vi "Camera.SetSession.vi"(8 "error in (no error)":errorcluster, 9 "Image":T1, 10 "Session":T2="cam0", 11 "Camera.Simulated":refnum<class "Camera.IMAQdx.lvclass">) -> (0 "error out":errorcluster, 3 "Camera.Simulated":refnum<class "Camera.IMAQdx.lvclass">)   [LabVIEW 2020, in "Camera.IMAQdx.lvclass"]
doc: "---------------------------------------------------------------\nJKI State Machine Objects™\nhttp://jki.net/state-machine-objects/\nCopyright (C) 2005-2015, JKI <info@jki.net>\nALL RIGHTS RESERVEDJKI State Machine Objects (SMO) 1.0.0.4\nJKI - JKI\nCopyright (c) 2015, JKI"
uses:
  Camera.IMAQdx.lvclass
  <vilib>/userdefined/High Color/IMAQdx.ctl
  <vilib>/vision/Image Controls.llb/IMAQ Image.ctl
  Camera.IMAQdx.lvclass/Camera.IMAQdx.ctl
panel:
  # "For instructions on how to use the JKI State Machine Objects, examples and video tutorials, visit:\nhttp://jki.net/state-machine-objects/\n\nJKI State Machine Objects™\nhttp://jki.net/state-machine-objects/\nCopyright (C) 2005-2015, JKI <info@jki.net>\nALL RIGHTS RESERVED"
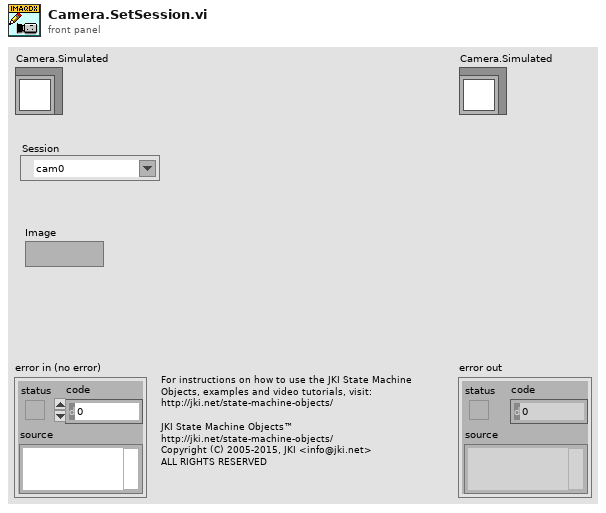
[diagram p1: front panel]
types:
  T1 = typedef "IMAQ Image.ctl" = refnum<image>
  T2 = typedef "IMAQdx.ctl" = refnum<k21>
  T3 = typedef "Camera.IMAQdx.lvclass/PrivateData--Ref.ctl" = refnum<data-value>
  T4 = typedef "Camera.IMAQdx.lvclass/PrivateData--Cluster.ctl" = cluster{"Session":T2, "Image":T1}
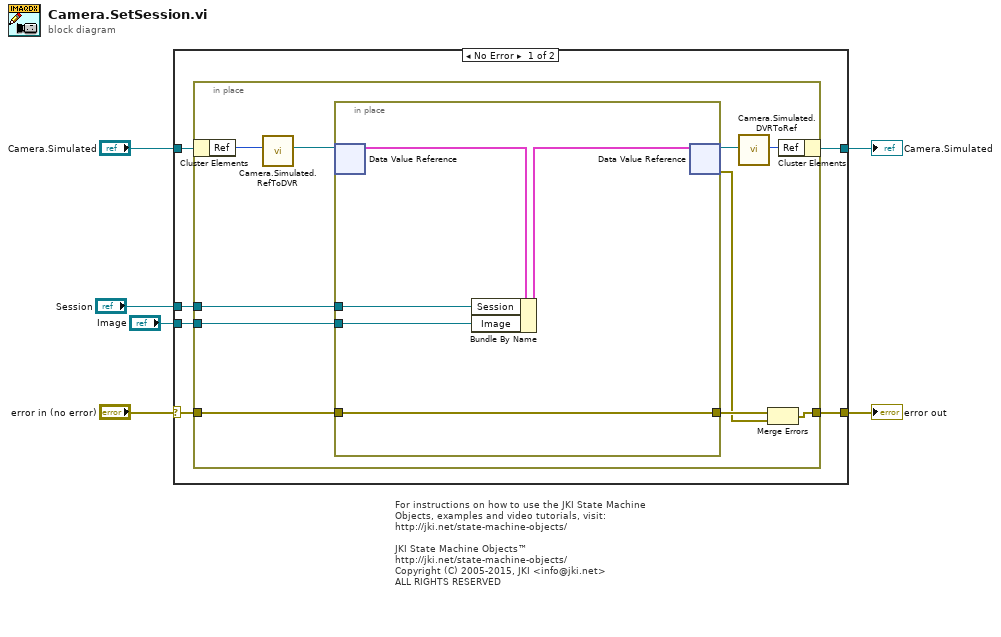
[diagram p0: block diagram]
diagram:
  # "For instructions on how to use the JKI State Machine Objects, examples and video tutorials, visit:\nhttp://jki.net/state-machine-objects/\n\nJKI State Machine Objects™\nhttp://jki.net/state-machine-objects/\nCopyright (C) 2005-2015, JKI <info@jki.net>\nALL RIGHTS RESERVED"
  n1 = case shown="No Error" "error in (no error)" {
    selector: "error in (no error)" -> [w10 w29]
    tunnel: [w9 w29] -> w5
    tunnel: [w11 w28] -> w6
    tunnel: "Camera.Simulated" -> [w12 w28]
    tunnel: "Session" -> [w8 _]
    tunnel: "Image" -> [w7 _]
    frame No Error {
      n2 = in-place {
        in-place-border: w10 -> [w22]
        in-place-border: [w19] -> w9
        in-place-border: w8 -> [w18]
        in-place-border: w7 -> [w13]
        n3 = in-place-cluster #1(w12) -> ("Ref"=w15:u32)
        n4 = call "Camera.Simulated.RefToDVR.vi"("Ref"=w15) -> ("Ref"=w14:T3)  [unwired: 10 in]
        n5 = in-place {
          in-place-border: w22 -> [w25]
          in-place-border: [w25] -> w21
          in-place-border: w18 -> [w24]
          in-place-border: w13 -> [w23]
          n6 = in-place-dvr #2(w14) -> (w27:T4)  [unwired: 1 out]
          n7 = Bundle By Name(cluster=w27, "Session"=w24, "Image"=w23) -> (w26:T4)
          n8 = in-place-dvr #2(w26) -> (w17:T3, w20:errorcluster)
        }
        n9 = call "Camera.Simulated.DVRToRef.vi"("Ref"=w17) -> ("Ref"=w16:u32)  [unwired: 10 in]
        n10 = Merge Errors(w21, w20) -> (w19:errorcluster)
        n11 = in-place-cluster #1("Ref"=w16) -> (w11:refnum<class "Camera.IMAQdx.lvclass">)
      }
    }
    frame Error {
    }
  }
  "error out" <- w5
  "Camera.Simulated" <- w6
